vi "Get Request Type.vi"(8 "error in (no error)":errorcluster, 11 "SetCurrentSceneCollection in":refnum<class "SetCurrentSceneCollection.lvclass">) -> (0 "error out":errorcluster, 2 "Request Type":string, 3 "SetCurrentSceneCollection out":refnum<class "SetCurrentSceneCollection.lvclass">)   [LabVIEW 2020, in "obs-websocket.lvlib" / "SetCurrentSceneCollection.lvclass"]
uses:
  SetCurrentSceneCollection.lvclass
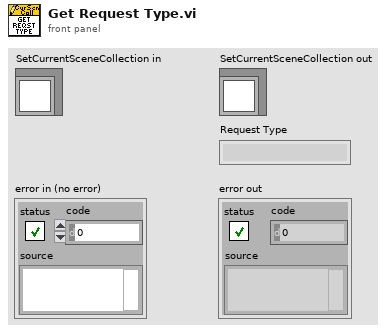
[diagram p1: front panel]
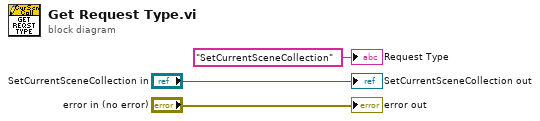
[diagram p0: block diagram]
diagram:
  "error out" <- "error in (no error)"
  "SetCurrentSceneCollection out" <- "SetCurrentSceneCollection in"
  "Request Type" <- "SetCurrentSceneCollection" ("Request Type")
